vi "JSON Array Size.vi"(8 "error in (no error)":errorcluster, 11 "JSON Tree In (JSON Array)":variant) -> (0 "error out":errorcluster, 2 "Array Size":i32, 3 "JSON Tree Passthrough (JSON Array)":variant)   [LabVIEW 2013, in "i3-json.lvlib"]
doc: "Use this template to build a VI to use as a subVI."
uses:
  i3-json.lvlib
  JSON Types/JSON Type.ctl
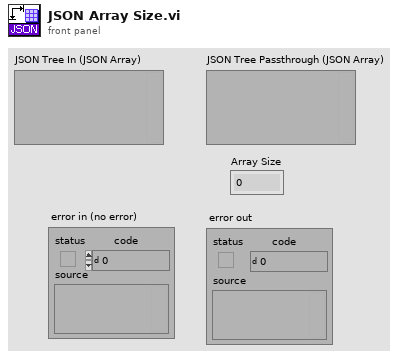
[diagram p1: front panel]
types:
  T1 = typedef "i3-json.lvlib/JSON Type.ctl" = enum8{"JSON Compatible", "JSON Array", "JSON Object", "JSON Null", "Double", "String", "Boolean", "Unknown", "Data JSON string"}
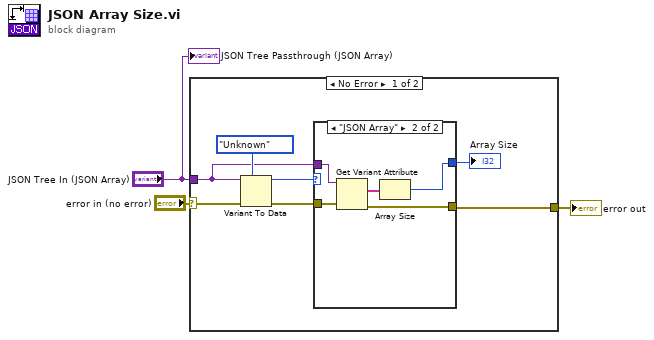
[diagram p0: block diagram]
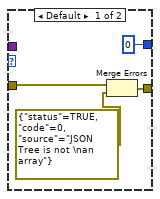
[diagram p2: hidden frame]
diagram:
  n1 = case shown="No Error" "error in (no error)" {
    selector: "error in (no error)" -> [w10 w20]
    tunnel: [w5 w20] -> w2
    tunnel: "JSON Tree In (JSON Array)" -> [w6 _]
    frame No Error {
      n2 = Variant To Data(error in=w10, type=JSON_Type."Unknown" ("JSON Type"), Variant=w6) -> (data=w8:T1, error out=w7:errorcluster)
      n3 = case shown="\"JSON Array\"" w8 {
        tunnel: w7 -> [w12 w19]
        tunnel: w6 -> [_ w18]
        tunnel: [w13 w17] -> w5
        tunnel: [0 w15] -> w4
        frame Default {
          n4 = Merge Errors(w12, errorcluster {"status"=TRUE, "code"=0, "source"="JSON Tree is not \nan array"} ("error out")) -> (w13:errorcluster)
        }
        frame "JSON Array" {
          n5 = Get Variant Attribute(Variant=w18, error in=w19) -> (names=w16:string[], error out=w17:errorcluster)  [unwired: 2 in, 2 out]
          n6 = Array Size(array=w16) -> (size(s)=w15:i32)
        }
      }
      "Array Size" <- w4
    }
    frame Error {
    }
  }
  "error out" <- w2
  "JSON Tree Passthrough (JSON Array)" <- "JSON Tree In (JSON Array)"
